vi "Mono Get Config.vi"(8 "error in (no error)":errorcluster, 11 "Mono In":refnum<class "Monochromator.lvclass">) -> (0 "error out":errorcluster, 3 "config data":T1)   [LabVIEW 2023, in "Examples.lvlib"]
doc: "This example shows how to retrieve the condifugration of the mono."
uses:
  Examples.lvlib
  Classes/Mono/configuration.ctl
  Classes/Mono/filterWheel.ctl
  Classes/Mono/grating.ctl
  Classes/Mono/mirror.ctl
  Classes/Mono/port.ctl
  Classes/Mono/Monochromator.lvclass
panel:
  # "Connector Pane"
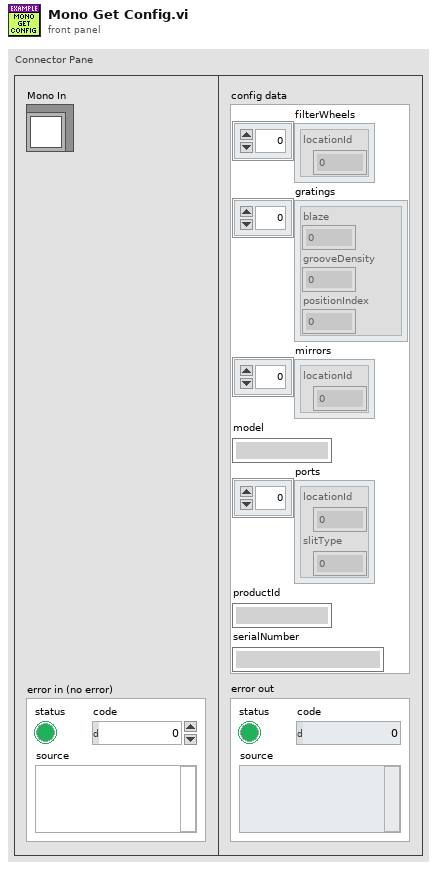
[diagram p1: front panel]
types:
  T1 = typedef "horiba.lvlib/Monochromator.lvclass/configuration.ctl" = cluster{"filterWheels":T2[], "gratings":T3[], "mirrors":T4[], "model":string, "ports":T5[], "productId":string, "serialNumber":string}
  T2 = typedef "horiba.lvlib/Monochromator.lvclass/filterWheel.ctl" = cluster{"locationId":i32}
  T3 = typedef "horiba.lvlib/Monochromator.lvclass/grating.ctl" = cluster{"blaze":i32, "grooveDensity":i32, "positionIndex":i32}
  T4 = typedef "horiba.lvlib/Monochromator.lvclass/mirror.ctl" = cluster{"locationId":i32}
  T5 = typedef "horiba.lvlib/Monochromator.lvclass/port.ctl" = cluster{"locationId":i32, "slitType":i32}
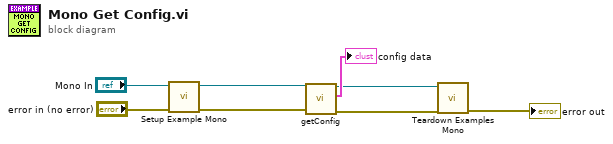
[diagram p0: block diagram]
diagram:
  n1 = call "Setup Example Mono.vi"("error in (no error)"="error in (no error)", "Mono In"="Mono In") -> ("error out"=w7:errorcluster, "Mono Out"=w8:refnum<class "Monochromator.lvclass">)  [unwired: 6 in, 2 out]
  n2 = call "getConfig.vi"("error in (no error)"=w7, "Monochromator in"=w8) -> ("error out"=w5:errorcluster, "config data"=→"config data":T1, "Monochromator out"=w1:refnum<class "Monochromator.lvclass">)  [unwired: 6 in, 1 out]
  n3 = call "Teardown Examples Mono.vi"("error in (no error)"=w5, "Monochromator in"=w1) -> ("error out"=→"error out":errorcluster)  [unwired: 9 in]
